vi "Stop Core.vi"(10 "final error code":i32, 11 "BNT_ULx-MCSV in":refnum<class "BNT_ULx-MCSV.lvclass">) -> (3 "BNT_ULx-MCSV out":refnum<class "BNT_ULx-MCSV.lvclass">)   [LabVIEW 2021, in "BNT_ULx.lvlib" / "BNT_ULx-MCSV.lvclass"]
doc: "(<B>Filename</B>: Actor Framework.lvlib:Actor.lvclass:Stop Core.vi)\n\nDefines what the actor does before it stops. Use the <B>final error code</B> input to determine whether the actor shut down in response to an error.\n\nBy default, this method does nothing. A descendant class may override it to define behavior, such as shutting down any processes the actor initiated in its override of the Actor Core method."
uses:
  BNT_ULx-MCSV.lvclass
  BNT_ULx-MCSV.lvclass/BNT_ULx-MCSV.ctl
  CSPP_Core/Actors/CSPP_DeviceActor/CSPP_DeviceActor.lvclass
  CSPP_Core/Classes/CSPP_ProcessVariables/PVConnection/PVConnection.lvclass
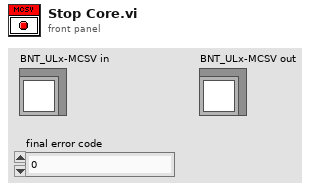
[diagram p1: front panel]
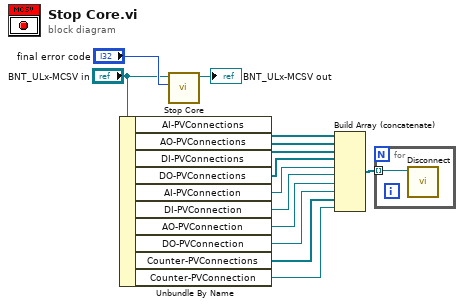
[diagram p0: block diagram]
diagram:
  n1 = Unbundle By Name("BNT_ULx-MCSV in") -> ("AI-PVConnections"=w12:refnum<class "PVConnection.lvclass">[], "AO-PVConnections"=w9:refnum<class "PVConnection.lvclass">[], "DI-PVConnections"=w8:refnum<class "PVConnection.lvclass">[], "DO-PVConnections"=w7:refnum<class "PVConnection.lvclass">[], "AI-PVConnection"=w6:refnum<class "PVConnection.lvclass">, "DI-PVConnection"=w5:refnum<class "PVConnection.lvclass">, "AO-PVConnection"=w4:refnum<class "PVConnection.lvclass">, "DO-PVConnection"=w3:refnum<class "PVConnection.lvclass">, "Counter-PVConnections"=w2:refnum<class "PVConnection.lvclass">[], "Counter-PVConnection"=w1:refnum<class "PVConnection.lvclass">)
  n2 = call-parent "Stop Core.vi"("final error code"="final error code", "CSPP_DeviceActor in"="BNT_ULx-MCSV in") -> ("CSPP_DeviceActor out"=→"BNT_ULx-MCSV out":refnum<class "BNT_ULx-MCSV.lvclass">)  [unwired: 9 in]
  n3 = Build Array (concatenate)(w12, w9, w8, w7, w6, w5, w4, w3, w2, w1) -> (w10:refnum<class "PVConnection.lvclass">[])
  n4 = for {
    tunnel: w10 -> [w15] mode=indexing
    n5 = call "Disconnect.vi"("PVConnection in"=w15) -> ()  [unwired: 9 in, 2 out]
  }
